vi "In_S6F1.vi"(8 "error in (no error)":errorcluster, 11 "S6 Message Class in":refnum<class "S6 Message Class.lvclass">) -> (0 "error out":errorcluster, 1 "OK?":bool, 2 "S6F1":T1, 3 "S6 Message Class out":refnum<class "S6 Message Class.lvclass">)   [LabVIEW 2020, in "SECS Communication.lvlib" / "S6 Message Class.lvclass"]
uses:
  S6 Message Class.lvclass
  D:/Dropbox/SECS/SECS_GEM v1.0.6/Com/SECS Communication/SECS-II Class/SECS-II Class.lvclass
  S6F1.ctl
  SECS-II Class/Format Code.ctl
  SECS-II Class/SECS-II Class.lvclass/SECS-II Class.ctl
  SECS-II Class/Variant To Data_U4.vi
  SECS-II Class/Variant To Data_ASCII.vi
  SECS-II Class/SECS-II Class.lvclass
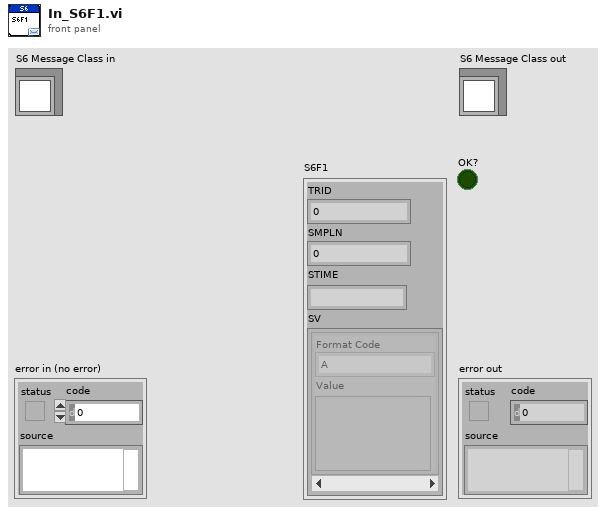
[diagram p1: front panel]
types:
  T1 = typedef "SECS Communication.lvlib/S6 Message Class.lvclass/S6F1.ctl" = cluster{"TRID":u32, "SMPLN":u32, "STIME":string, "SV":cluster{"Format Code":T2, "Value":variant}[]}
  T2 = typedef "SECS Communication.lvlib/SECS-II Class.lvclass/Format Code.ctl" = enum16{"L", "A", "B", "Boolean", "J", "I1", "I2", "I4", "I8", "U1", "U2", "U4", "U8", "F4", "F8", "Char"}
  T3 = typedef "SECS Communication.lvlib/SECS-II Class.lvclass/Message Data.ctl" = cluster{"Index":i32, "Data Item Format":T4, "Format Code":T2, "Parent Index":i32, "Child Index":i32[], "Data":variant}
  T4 = typedef "SECS Communication.lvlib/SECS-II Class.lvclass/Data Item Format.ctl" = enum16{"Data Type", "Value"}
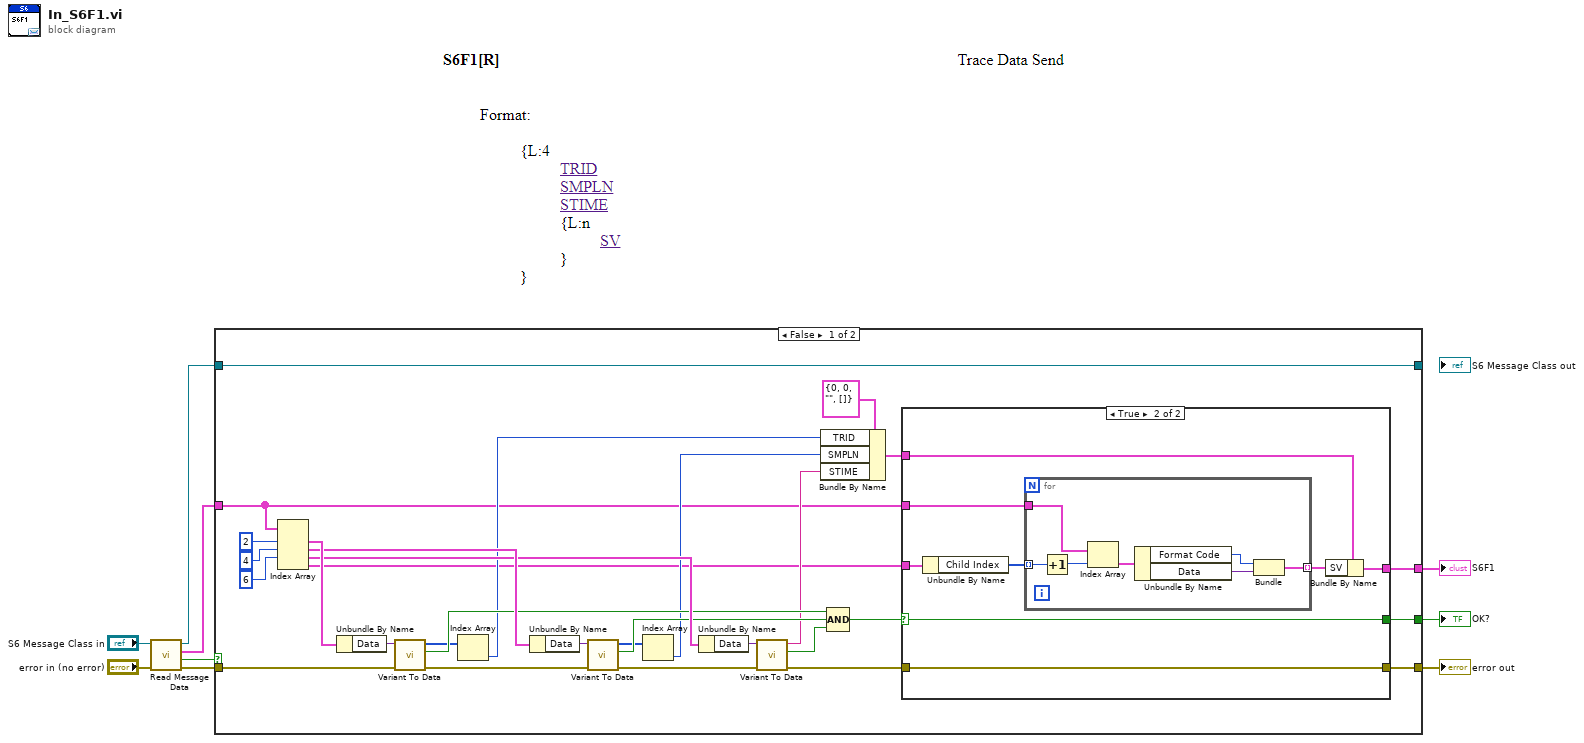
[diagram p0: block diagram]
diagram:
  n1 = call "Read Message Data.vi"("error in (no error)"="error in (no error)", "SECS-II Class in"="S6 Message Class in") -> ("error out"=w8:errorcluster, "Empty?"=w7:bool, "Message Data"=w9:T3[], "SECS-II Class out"=w6:refnum<class "S6 Message Class.lvclass">)  [unwired: 6 in]
  n2 = case shown="False" w7 {
    tunnel: w9 -> [w14 _]
    tunnel: w8 -> [w36 w57]
    tunnel: [w12 w57] -> w4
    tunnel: w6 -> [w35 w58]
    tunnel: [w35 w58] -> _
    tunnel: [w11 _] -> w5
    tunnel: [w10 _] -> w3
    frame False {
      n3 = Index Array(array=w14, index #1=2 ("index"), index #2=4 ("index"), index #3=6 ("index")) -> (element #1=w38:T3, element #2=w30:T3, element #3=w27:T3, element #4=w15:T3)  [unwired: 1 in]
      n4 = Unbundle By Name(w38) -> ("Data"=w37:variant)
      n5 = call-poly "Variant To Data.vi"("error in (no error)"=w36, "Variant"=w37) -> ("error out"=w31:errorcluster, "OK?"=w26:bool, "Data"=w23:u32[])  [unwired: 7 in]
      n6 = Index Array(array=w23) -> (element=w20:u32)  [unwired: 1 in]
      n7 = Unbundle By Name(w30) -> ("Data"=w32:variant)
      n8 = call-poly "Variant To Data.vi"("error in (no error)"=w31, "Variant"=w32) -> ("error out"=w28:errorcluster, "OK?"=w25:bool, "Data"=w22:u32[])  [unwired: 7 in]
      n9 = Index Array(array=w22) -> (element=w19:u32)  [unwired: 1 in]
      n10 = Unbundle By Name(w27) -> ("Data"=w29:variant)
      n11 = call-poly "Variant To Data.vi"("error in (no error)"=w28, "Variant"=w29) -> ("error out"=w16:errorcluster, "OK?"=w24:bool, "Data"=w18:string)  [unwired: 7 in]
      n12 = Bundle By Name(cluster=T1 {"TRID"=0, "SMPLN"=0, "STIME"="", "SV"=[]} ("S6F1"), "TRID"=w20, "SMPLN"=w19, "STIME"=w18) -> (w13:T1)
      n13 = Compound Arithmetic op=AND(w26, w25, w24) -> (w17:bool)
      n14 = case shown="True" w17 {
        selector: w17 -> [w41 w42]
        tunnel: w16 -> [w40 w44]
        tunnel: w15 -> [_ w49]
        tunnel: w14 -> [_ w47]
        tunnel: w13 -> [_ w46]
        tunnel: [w40 w44] -> w12
        tunnel: [_ w43] -> w11
        tunnel: [w41 w42] -> w10
        frame False {
        }
        frame True {
          n15 = Unbundle By Name(w49) -> ("Child Index"=w48:i32[])
          n16 = for {
            tunnel: w48 -> [w56] mode=indexing
            tunnel: w47 -> [w55]
            tunnel: [w50] -> w45 mode=indexing
            n17 = Increment(x=w56) -> (x+1=w54:i32)
            n18 = Index Array(array=w55, index=w54) -> (element=w53:T3)
            n19 = Unbundle By Name(w53) -> ("Format Code"=w51:T2, "Data"=w52:variant)
            n20 = Bundle("Format Code"=w51, "Data"=w52) -> (w50:cluster{"Format Code":T2, "Data":variant})  [unwired: 1 in]
          }
          n21 = Bundle By Name(cluster=w46, "SV"=w45) -> (w43:T1)
        }
      }
    }
    frame True {
    }
  }
  "error out" <- w4
  "S6F1" <- w5
  "OK?" <- w3
